vi "RSZVB Instrument Options.vi"(8 "error in (no error)":errorcluster {"code" format="%.0x"}, 11 "VISA session":refnum<visa-resource-name>) -> (0 "error out":errorcluster {"code" format="%.0x"}, 1 "Options List":string, 2 "Instrument Version":string, 3 "dup VISA session":refnum<visa-resource-name>, 4 "Ports":i32, 5 "Model":string, 6 "Version":T1)   [LabVIEW 2015]
doc: "This VI returns the instrument version number and the list of options which the instrument is equipped with.\n\nRemote-control command(s):\n*OPT?"
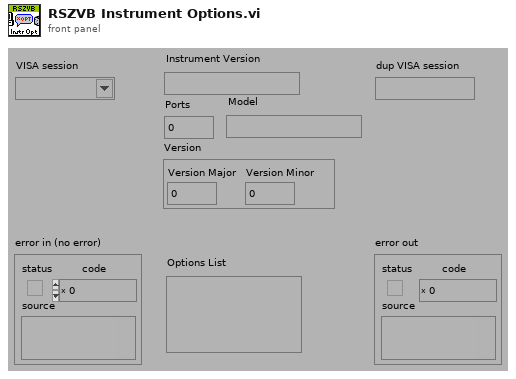
[diagram p1: front panel]
types:
  T1 = cluster{"Version Major":i32, "Version Minor":i32}
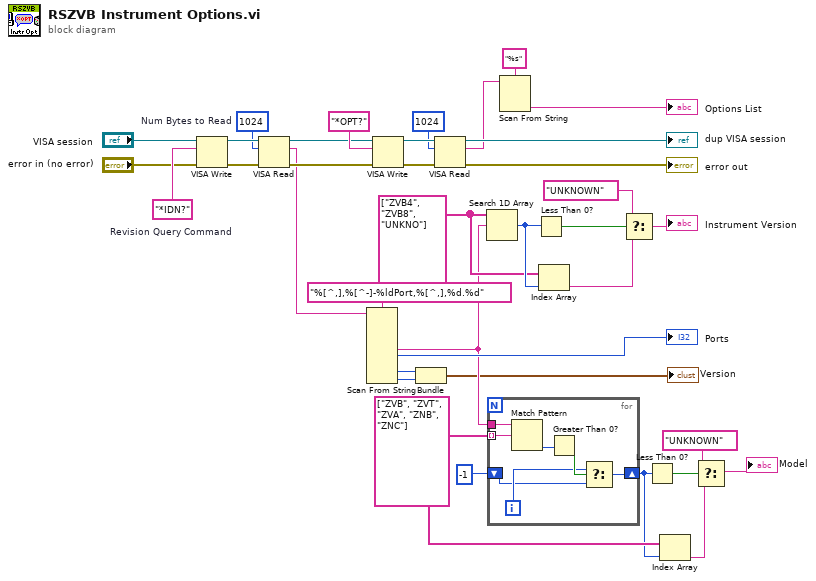
[diagram p0: block diagram]
diagram:
  w11 = string[] ["ZVB", "ZVT", "ZVA", "ZNB", "ZNC"]
  w15 = string[] ["ZVB4", "ZVB8", "UNKNO"]
  w37 = "*IDN?"  # Revision Query Command
  w34 = u32 1024  # Num Bytes to Read
  n1 = VISA Write(VISA resource name="VISA session", write buffer=w37, error in (no error)="error in (no error)") -> (VISA resource name out=w35:refnum<visa-resource-name>, error out=w36:errorcluster)  [unwired: 1 out]
  n2 = VISA Read(VISA resource name=w35, byte count=w34, error in (no error)=w36) -> (VISA resource name out=w26:refnum<visa-resource-name>, read buffer=w4:string, error out=w27:errorcluster)  [unwired: 1 out]
  n3 = Scan From String(format string="%[^,],%[^-]-%ldPort,%[^,],%d.%d", input string=w4) -> (output 2=w5:string, output 3=→"Ports":i32, output 5=w3:i32, output 6=w2:i32)  [unwired: 10 in, 3 out]
  n4 = VISA Write(VISA resource name=w26, write buffer="*OPT?", error in (no error)=w27) -> (VISA resource name out=w29:refnum<visa-resource-name>, error out=w30:errorcluster)  [unwired: 1 out]
  n5 = Bundle(w3, w2) -> (→"Version":cluster{i32, i32})  [unwired: 1 in]
  n6 = VISA Read(VISA resource name=w29, byte count=u32 1024, error in (no error)=w30) -> (VISA resource name out=→"dup VISA session":refnum<visa-resource-name>, read buffer=w23:string, error out=→"error out":errorcluster)  [unwired: 1 out]
  n7 = Search 1D Array(1D array=w15, element=w5) -> (index of element=w19:i32)  [unwired: 1 in]
  n8 = for {
    tunnel: w11 -> [w44] mode=indexing
    tunnel: w5 -> [w43]
    shift-right: [w40] -> w9
    shift-left: -1 -> [w38]
    i -> [w39]
    n9 = Match Pattern(string=w43, regular expression=w44) -> (offset past match=w42:i32)  [unwired: 1 in, 3 out]
    n10 = Greater Than 0?(x=w42) -> (x > 0?=w41:bool)
    n11 = Select(t=w39, s=w41, f=w38) -> (s? t:f=w40:i32)
  }
  n12 = Scan From String(format string="%s", input string=w23) -> (output 1=→"Options List":string)  [unwired: 3 in, 3 out]
  n13 = Less Than 0?(x=w19) -> (x < 0?=w20:bool)
  n14 = Index Array(array=w15, index=w19) -> (element=w18:string)
  n15 = Select(t="UNKNOWN", s=w20, f=w18) -> (s? t:f=→"Instrument Version":string)
  n16 = Less Than 0?(x=w9) -> (x < 0?=w10:bool)
  n17 = Index Array(array=w11, index=w9) -> (element=w7:string)
  n18 = Select(t="UNKNOWN", s=w10, f=w7) -> (s? t:f=→"Model":string)
